vi "Get Fiducial.vi"(6 "error in":errorcluster, 7 "Fiducial Type":string, 9 "CameraTool Class In":refnum<class "CameraTool Class.lvclass">) -> (0 "error out":errorcluster, 1 "Fiducial Image Position":refnum<class "Vec3d Class.lvclass">, 3 "CameraTool Class Out":refnum<class "CameraTool Class.lvclass">)   [LabVIEW 2011, in "CameraTool Class.lvclass"]
doc: "This VI looks for fiducials in input images. It returns the number of fiducials found in the input image and a list of up to 10 x,y pairs of fiducial locations in the image"
uses:
  CameraTool Class.lvclass
  Vec3d Class/Vec3d Class.lvclass
  Gantry Class/Gantry Class.lvclass
  <vilib>/Utility/config.llb/Read Key (Double).vi
  <vilib>/Utility/config.llb/NI_LVConfig.lvlib
  gVision/Release/gVision.dll
panel:
  in  "interactive":bool
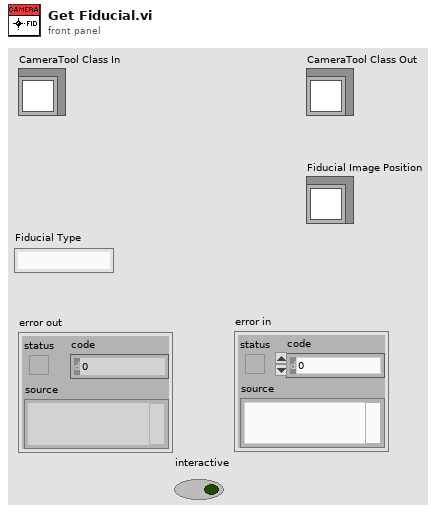
[diagram p1: front panel]
types:
  T1 = enum32{"Map Pixel Pointer", "Unmap Pixel Pointer", "Get Pixels Infos"}
  T2 = typedef "IMAQ Image.ctl" = refnum<image>
  T3 = typedef "NI_LVConfig.lvlib/Config Data RefNum.ctl" = refnum<k1>
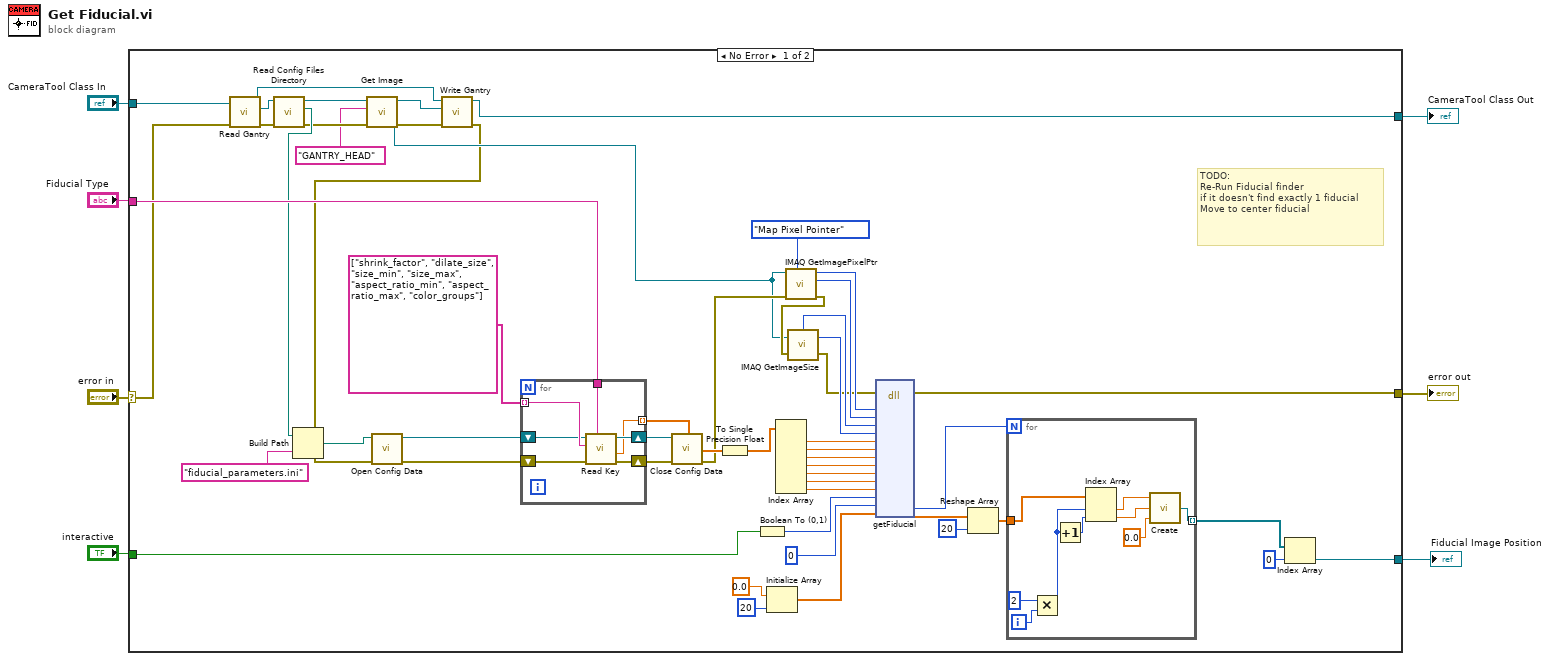
[diagram p0: block diagram]
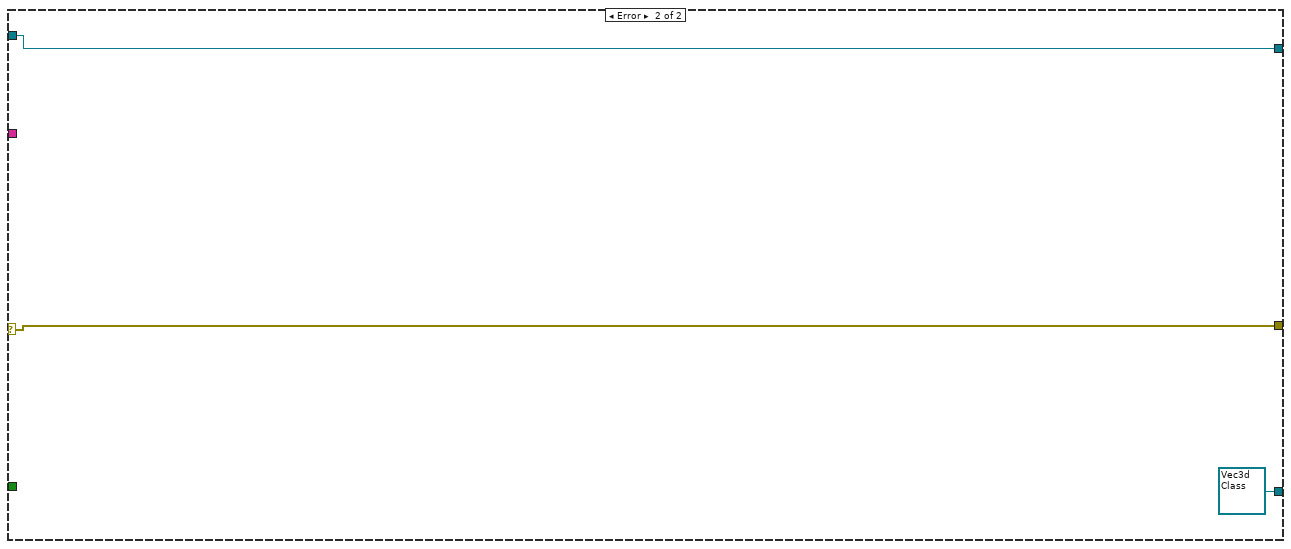
[diagram p2: hidden frame]
diagram:
  n1 = case shown="No Error" "error in" {
    selector: "error in" -> [w21 w79]
    tunnel: [w11 w79] -> w6
    tunnel: "CameraTool Class In" -> [w29 w78]
    tunnel: "Fiducial Type" -> [w28 _]
    tunnel: [w16 w78] -> w3
    tunnel: "interactive" -> [w15 _]
    tunnel: [w8 refnum<class "Vec3d Class.lvclass"> refnum ("Vec3d Class out")] -> w1
    frame No Error {
      # "TODO:\nRe-Run Fiducial finder\nif it doesn't find exactly 1 fiducial\nMove to center fiducial"
      n2 = call-dynamic "Read Gantry.vi"("error in (no error)"=w21, "Tool Class in"=w29) -> ("error out"=w26:errorcluster, "Gantry Class.lvclass"=w27:refnum<class "Gantry Class.lvclass">, "Tool Class out"=w20:refnum<class "CameraTool Class.lvclass">)  [unwired: 7 in]
      n3 = call-dynamic "Read Config Files Directory.vi"("error in (no error)"=w26, "Gantry Class in"=w27) -> ("error out"=w22:errorcluster, "Config Files Directory"=w25:path, "Gantry Class out"=w24:refnum<class "Gantry Class.lvclass">)  [unwired: 7 in]
      n4 = Build Path(base path=w25, name or relative path="fiducial_parameters.ini") -> (appended path=w47:path)
      n5 = call "Get Image.vi"("error in (no error)"=w22, "Camera Name"="GANTRY_HEAD", "Gantry Class in"=w24) -> ("error out"=w18:errorcluster, "Image Out"=w23:T2, "Gantry Class out"=w19:refnum<class "Gantry Class.lvclass">)  [unwired: 6 in]
      n6 = call-dynamic "Write Gantry.vi"("error in (no error)"=w18, "Gantry Class.lvclass"=w19, "Tool Class in"=w20) -> ("error out"=w17:errorcluster, "Tool Class out"=w16:refnum<class "CameraTool Class.lvclass">)  [unwired: 7 in]
      n7 = call <vilib>:"Open Config Data.vi"("error in (no error)"=w17, "configuration file path"=w47) -> ("error out"=w45:errorcluster, "refnum"=w44:T3)  [unwired: 7 in, 1 out]
      n8 = for {
        tunnel: string[] ["shrink_factor", "dilate_size", "size_min", "size_max", "aspect_ratio_min", "aspect_ratio_max", "color_groups"] -> [w76] mode=indexing
        tunnel: w28 -> [w75]
        shift-right: [w73] -> w31
        shift-left: w45 -> [w74]
        shift-right: [w71] -> w32
        shift-left: w44 -> [w72]
        tunnel: [w70] -> w43 mode=indexing
        n9 = call-poly <vilib>:"Read Key.vi"("section"=w75, "error in (no error)"=w74, "key"=w76, "refnum"=w72) -> ("error out"=w73:errorcluster, "value"=w70:dbl, "refnum out"=w71:T3)  [unwired: 4 in, 1 out]
      }
      n10 = call <vilib>:"Close Config Data.vi"("error in (no error)"=w31, "refnum"=w32) -> ("error out"=w30:errorcluster)  [unwired: 8 in, 1 out]
      n11 = To Single Precision Float(number=w43) -> (single precision float=w42:sgl[])
      n12 = Boolean To (0,1)(Boolean=w15) -> (0, 1=w49:i16)
      n13 = Initialize Array(0.0 ("element"), 20 ("dimension size")) -> (w56:dbl[])
      n14 = Index Array(array=w42) -> (element #1=w41:sgl, element #2=w40:sgl, element #3=w39:sgl, element #4=w38:sgl, element #5=w37:sgl, element #6=w36:sgl, element #7=w35:sgl)  [unwired: 7 in]
      n15 = call "IMAQ GetImagePixelPtr"("Function"=T1."Map Pixel Pointer", "error in (no error)"=w30, "Image"=w23) -> ("error out"=w34:errorcluster, "LineWidth(Pixels)"=w52:i32, "Pixel Pointer out"=w51:u64)  [unwired: 3 in, 3 out]
      n16 = call "IMAQ GetImageSize"("Image"=w23, "error in (no error)"=w34) -> ("Y Resolution"=w54:i32, "X Resolution"=w53:i32, "error out"=w33:errorcluster)  [unwired: 2 in]
      n17 = dll-call lib="C:/Users/Husker/Desktop/gantry/gVision/Release/gVision.dll" fn="getFiducial"(error in=w33, "imgPtr"=w51, "imgLineWidth"=w52, "imgWidth"=w53, "imgHeight"=w54, "shrinkFactor"=w41, "dilateSize"=w40, "sizeMin"=w39, "sizeMax"=w38, "arMin"=w37, "arMax"=w36, "colorGroups"=w35, "interactive"=w49, "numFiducials"=0, "coords"=w56) -> (error out=w11:errorcluster, "numFiducials"=w13:i32, "coords"=w59:sgl[])  [unwired: 15 in, 1 out]
      n18 = Reshape Array(w59, 20 ("dimension size")) -> (w12:sgl[])
      n19 = for {
        N: w13 -> [_]
        tunnel: w12 -> [w69]
        tunnel: [w61] -> w9 mode=indexing
        i -> [w68]
        n20 = Multiply(x=2, y=w68) -> (x*y=w66:i32)
        n21 = Increment(x=w66) -> (x+1=w65:i32)
        n22 = Index Array(array=w69, index #1=w66, index #2=w65) -> (element #1=w64:sgl, element #2=w63:sgl)
        n23 = call "Create.vi"("Z"=0.0, "Y"=w63, "X"=w64) -> ("Vec3d Class out"=w61:refnum<class "Vec3d Class.lvclass">)
      }
      n24 = Index Array(array=w9, index=0) -> (element=w8:refnum<class "Vec3d Class.lvclass">)
    }
    frame Error {
    }
  }
  "error out" <- w6
  "CameraTool Class Out" <- w3
  "Fiducial Image Position" <- w1
